vi "Modbus Write STR8.vi"(7 "Slave Address":u8, 8 "error in (no error)":errorcluster, 9 "Input String (8 chars)":string, 10 "Register Start Address":u16 format="%x", 11 "VISA resource in":refnum<visa-resource-name>) -> (0 "error out":errorcluster, 3 "VISA resource out":refnum<visa-resource-name>)   [LabVIEW 2023, in "Voegtlin_NI_SMART_Modbus_Drivers.lvlib"]
doc: "Schreibe einen String mit 8 Zeichen an die angegebene Startadresse des selektierten Geraetes. Es werden immer 8 Zeichen geschrieben, unabhaengig von der Laenge des uebergebenen Strings. Überschuessige Zeichen werden ignoriert, fehlende durch leere Platzhalter ergaenzt.\nEs werden insgesammt 4 Register geschrieben.\nDer COM-Port muss dazu initialisiert sein (benutze\" Modbus Init.vi\")."
uses:
  Voegtlin_NI_SMART_Modbus_Drivers.lvlib
  Enums/Modbus Comm.ctl
panel:
  out "U16 input data to write\n(array)":u16[](array[numeric])
  # "Input Data"
  # "Internal Data"
  # "Output Data"
  # "(Inputmaske in HEX)"
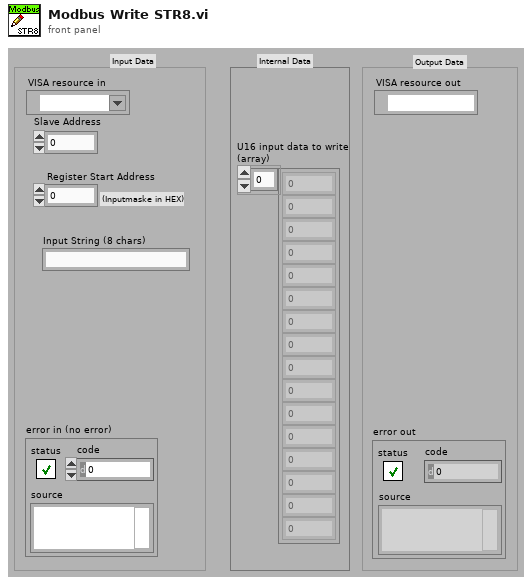
[diagram p1: front panel]
types:
  T1 = typedef "Voegtlin_NI_SMART_Modbus_Drivers.lvlib/Modbus Comm.ctl" = enum16{"Init", "Read", "Write", "Exit"}
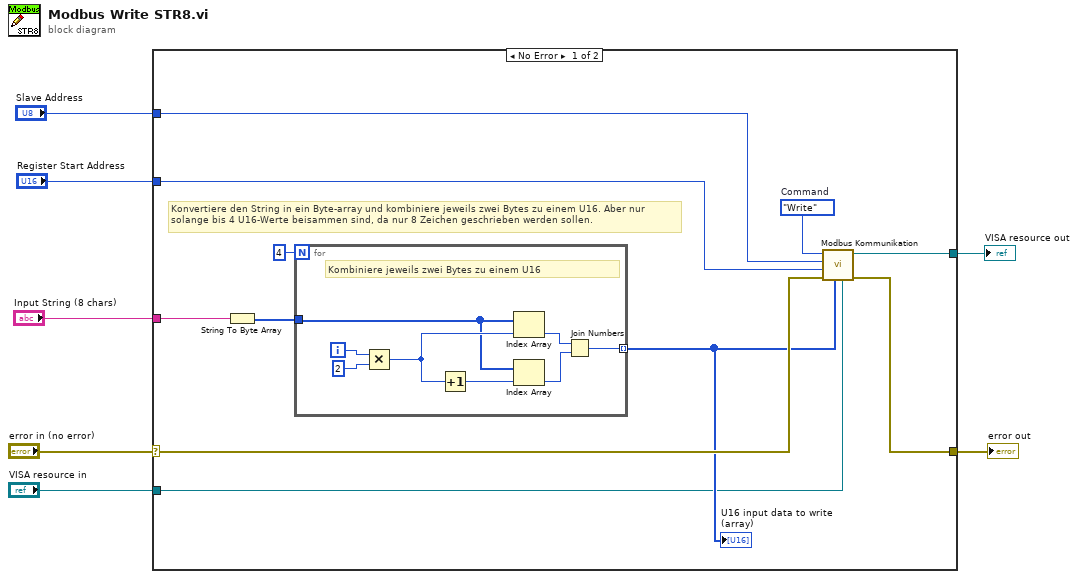
[diagram p0: block diagram]
diagram:
  n1 = case shown="No Error" "error in (no error)" {
    selector: "error in (no error)" -> [w13 w28]
    tunnel: [w17 w28] -> w7
    tunnel: "Register Start Address" -> [w11 _]
    tunnel: "Input String (8 chars)" -> [w16 _]
    tunnel: "Slave Address" -> [w10 _]
    tunnel: "VISA resource in" -> [w9 w27]
    tunnel: [w8 w27] -> w1
    frame No Error {
      w18 = Modbus_Comm."Write"  # Command
      # "Konvertiere den String in ein Byte-array und kombiniere jeweils zwei Bytes zu einem U16. Aber nur solange bis 4 U16-Werte beisammen sind, da nur 8 Zeichen geschrieben werden sollen."
      n2 = String To Byte Array(string=w16) -> (unsigned byte array=w15:u8[])
      n3 = for {
        N: 4 -> [_]
        tunnel: w15 -> [w22]
        tunnel: [w19] -> w12 mode=indexing
        i -> [w25]
        # "Kombiniere jeweils zwei Bytes zu einem U16"
        n4 = Multiply(x=w25, y=2 ("x")) -> (x*y=w24:i32)
        n5 = Increment(x=w24) -> (x+1=w23:i32)
        n6 = Index Array(array=w22, index=w24) -> (element=w21:u8)
        n7 = Index Array(array=w22, index=w23) -> (element=w20:u8)
        n8 = Join Numbers(hi=w21, lo=w20) -> ((hi.lo)=w19:u16)
      }
      "U16 input data to write\n(array)" <- w12
      n9 = call "Modbus Kommunikation.vi"("VISA resource in"=w9, "Data In / #Reads [U16]"=w12, "error in (no error)"=w13, "Register Start Address"=w11, "Slave Address"=w10, "Command"=w18) -> ("error out"=w17:errorcluster, "VISA resource out"=w8:refnum<visa-resource-name>)  [unwired: 3 in, 1 out]
    }
    frame Error {
    }
  }
  "error out" <- w7
  "VISA resource out" <- w1
